vi "FP_to_DSC.vi"(6 "Mode":u16, 7 "Enum":enum16{"CF", "MNK"}(ring), 8 "FP Status Bits":u32[](array[numeric]), 9 "PT Data":dbl[](array[numeric]), 10 "MG Data":dbl[](array[numeric]), 11 "FP Data":sgl[](array[numeric])) -> ()   [LabVIEW 2013]
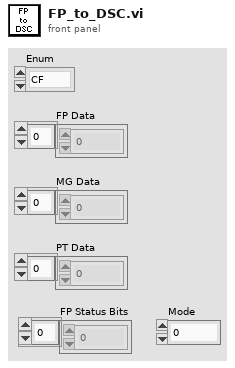
[diagram p1: front panel]
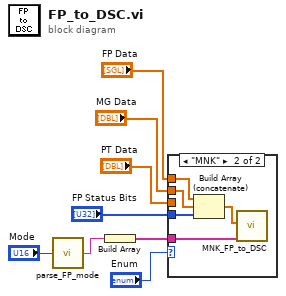
[diagram p0: block diagram]
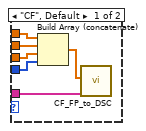
[diagram p2: hidden frame]
diagram:
  n1 = call "parse_FP_mode.vi"("line index"="Mode") -> ("output string"=w7:string)
  n2 = Build Array(w7) -> (w8:string[])
  n3 = case shown="\"MNK\"" "Enum" {
    tunnel: "FP Data" -> [w13 w19]
    tunnel: "MG Data" -> [w12 w18]
    tunnel: "PT Data" -> [w11 _]
    tunnel: w8 -> [w10 w15]
    tunnel: "FP Status Bits" -> [w9 w17]
    frame "CF", Default {
      n4 = Build Array (concatenate)(w13, w12, w11, w9) -> (w14:dbl[])
      n5 = call "CF_FP_to_DSC.vi"("str"=w10, "dbl"=w14) -> ()  [unwired: 2 in]
    }
    frame "MNK" {
      n6 = Build Array (concatenate)(w19, w18, w17) -> (w16:dbl[])
      n7 = call "MNK_FP_to_DSC.vi"("str"=w15, "dbl"=w16) -> ()  [unwired: 2 in]
    }
  }
